vi "convertToDAC.vi"(8 "error in (no error)":errorcluster, 10 "Voltage":dbl[unit], 11 "ILC in":refnum<class "ILC.lvclass">) -> (0 "error out":errorcluster, 2 "Counts":u16, 3 "ILC out":refnum<class "ILC.lvclass">)   [LabVIEW 2015, in "ILCCommon.lvlib" / "ILC.lvclass"]
uses:
  <userlib>/Common/ILC/ILC/ILC.lvclass
  <userlib>/Common/ILC/ILC/ILC.lvclass/ILC.ctl
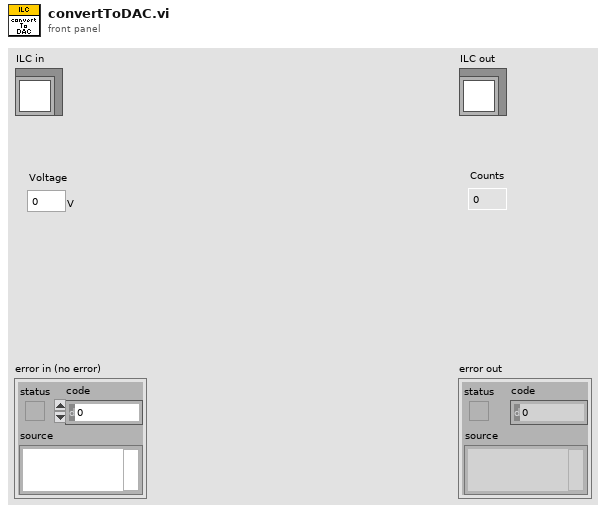
[diagram p1: front panel]
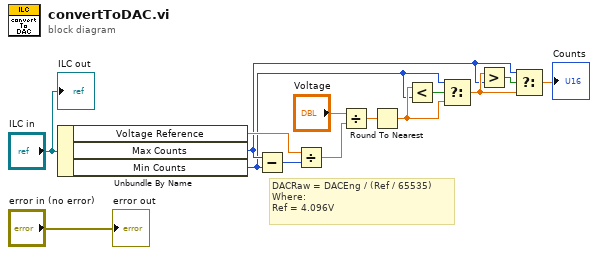
[diagram p0: block diagram]
diagram:
  # "DACRaw = DACEng / (Ref / 65535)\nWhere:\nRef = 4.096V"
  n1 = Unbundle By Name("ILC in") -> ("Voltage Reference"=w11:dbl[unit], "Max Counts"=w3:i32, "Min Counts"=w2:i32)
  n2 = Subtract(x=w3, y=w2) -> (x-y=w12:i32)
  n3 = Divide(x=w11, y=w12) -> (x/y=w10:dbl[unit])
  n4 = Divide(x="Voltage", y=w10) -> (x/y=w8:dbl)
  n5 = Round To Nearest(number=w8) -> (nearest integer value=w4:dbl)
  n6 = Less?(x=w4, y=w2) -> (x < y?=w7:bool)
  n7 = Select(t=w2, s=w7, f=w4) -> (s? t:f=w6:dbl)
  n8 = Greater?(x=w6, y=w3) -> (0:w5:bool)
  n9 = Select(t=w3, s=w5, f=w6) -> (s? t:f=→"Counts":dbl)
  "error out" <- "error in (no error)"
  "ILC out" <- "ILC in"
